vi "Read Water Level Actor.vi"(11 "Simulated Cooler":refnum<class "Simulated Evaporative Cooler.lvclass">) -> (2 "Water Level":refnum<class "Water Level.lvclass">)   [LabVIEW 2025, in "Simulated Evaporative Cooler.lvclass"]
uses:
  Simulated Evaporative Cooler.lvclass
  Water Level/Water Level.lvclass
  Simulated Water Level/Simulated Water Level.lvclass
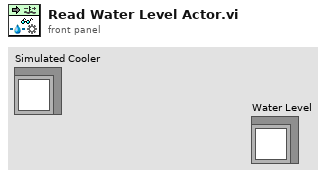
[diagram p1: front panel]
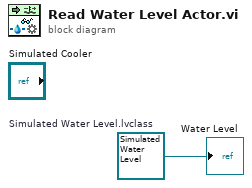
[diagram p0: block diagram]
diagram:
  w1 = refnum<class "Simulated Water Level.lvclass"> refnum  # Simulated Water Level.lvclass
  "Water Level" <- w1
